vi "Model.vi"() -> ()   [LabVIEW 2016]
uses:
  <vilib>/Analysis/Matrix/Datatypes/RealMatrix.ctl
  Enum_activations.ctl
  <vilib>/Analysis/Matrix/NI_Matrix.lvlib
panel:
  out "Cost":dbl(graph)
  in  "Learning_Rate":dbl
  out "m":i32
  out "Costs":dbl[](array[numeric])
  in  "Y":T1
  in  "Parameters":T3(array[cluster])
  in  "Epochs":i32
  out "Predictions":T1
  in  "X":T1
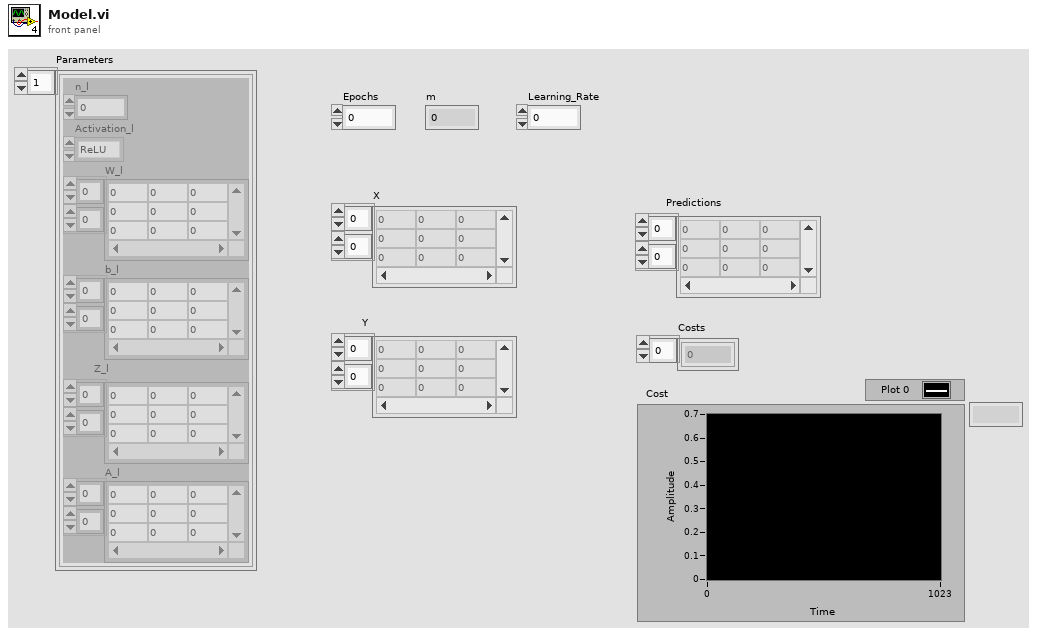
[diagram p1: front panel]
types:
  T1 = typedef "NI_Matrix.lvlib/RealMatrix.ctl" = dbl[][]
  T2 = typedef "Enum_activations.ctl" = enum16{"ReLU", "Sigmoid"}
  T3 = cluster{"n_l":i32, "Activation_l":T2, "W_l":T1, "b_l":T1, "Z_l":T1, "A_l":T1}[]
  T4 = cluster{"n_l":i32, "Activation_l":T2, "W_l":T1, "b_l":T1, "Z_l":T1, "A_l":T1}
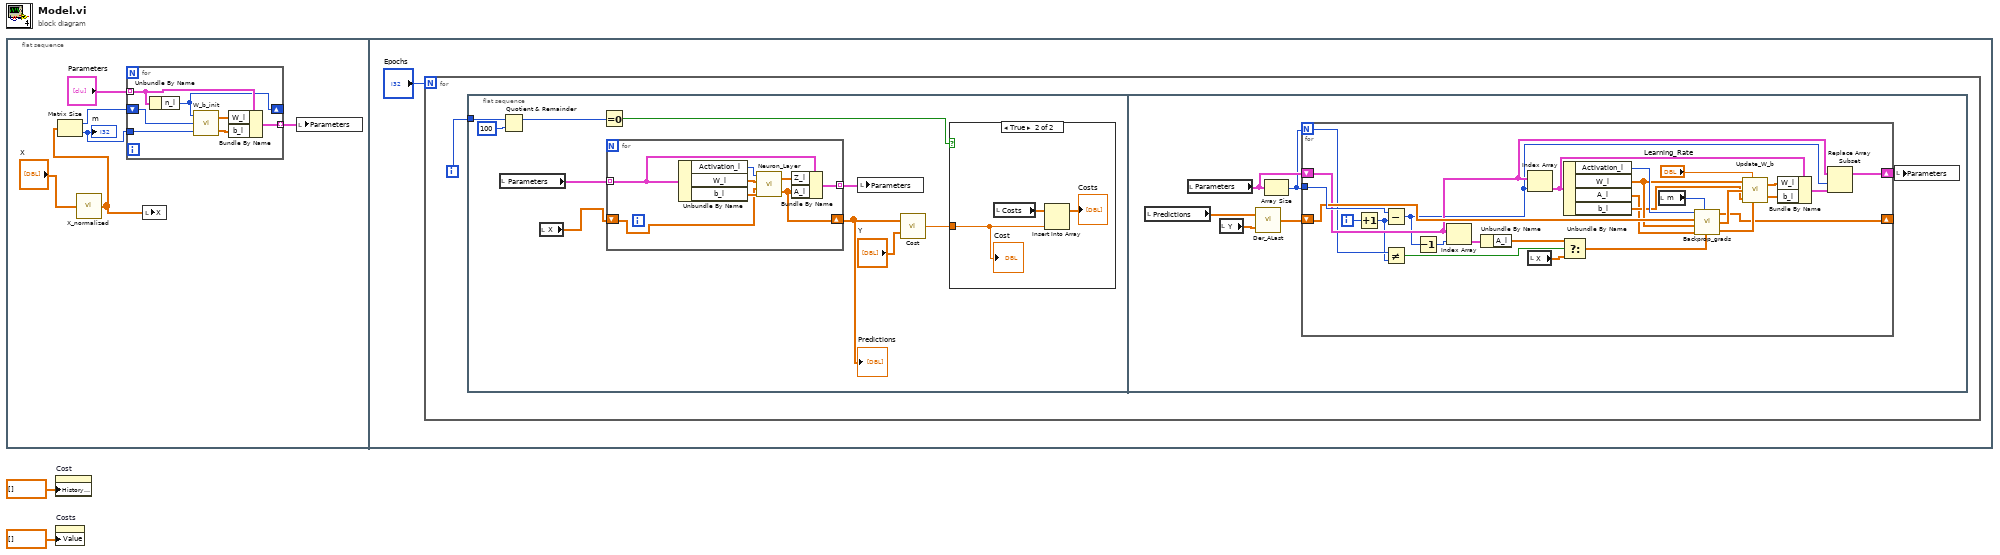
[diagram p0: block diagram]
diagram:
  n1 = flat-sequence {
    frame #0 {
      n2 = call "X_normalized.vi"("X"="X") -> ("X_normalized"=w3:T1)
      n3 = Matrix Size(0:w3) -> (1:w5:i32, 2:w6:i32)
      "m" <- w6
      n4 = for {
        tunnel: "Parameters" -> [w14] mode=indexing
        tunnel: w6 -> [w15]
        shift-right: [w10] -> _
        shift-left: w5 -> [w9]
        tunnel: [w11] -> w7 mode=indexing
        n5 = Unbundle By Name(w14) -> ("n_l"=w10:i32)
        n6 = call "W_b_init.vi"("m"=w15, "n_l-1"=w9, "n_l"=w10) -> ("b_l"=w12:T1, "W_l"=w13:T1)
        n7 = Bundle By Name(cluster=w14, "W_l"=w13, "b_l"=w12) -> (w11:T4)
      }
      n8 = local write "X"(w3) -> ()
      n9 = local write "Parameters"(w7) -> ()
    }
    frame #1 {
      n10 = for {
        N: "Epochs" -> [_]
        i -> [w17]
        n11 = flat-sequence {
          tunnel: w17 -> [w25]
          frame #0 {
            n12 = local read "Parameters"() -> (w27:T3)
            n13 = Quotient & Remainder(x=w25, y=100) -> (x-y*floor(x/y)=w23:i32)  [unwired: 1 out]
            n14 = local read "X"() -> (w18:T1)
            n15 = Equal To 0?(x=w23) -> (x = 0?=w22:bool)
            n16 = for {
              tunnel: w27 -> [w35] mode=indexing
              shift-right: [w33] -> w19
              shift-left: w18 -> [w31]
              tunnel: [w32] -> w20 mode=indexing
              n17 = Unbundle By Name(w35) -> ("Activation_l"=w38:T2, "W_l"=w37:T1, "b_l"=w36:T1)
              n18 = call "Neuron_Layer.vi"("b"=w36, "A_l-1"=w31, "W"=w37, "Activation"=w38) -> ("A_l"=w33:T1, "Z"=w34:T1)
              n19 = Bundle By Name(cluster=w35, "Z_l"=w34, "A_l"=w33) -> (w32:T4)
            }
            "Predictions" <- w19
            n20 = local write "Parameters"(w20) -> ()
            n21 = call "Cost.vi"("Y"="Y", "Predictions"=w19) -> ("Cost"=w21:dbl)
            n22 = case shown="True" w22 {
              tunnel: w21 -> [_ w28]
              frame False {
              }
              frame True {
                n23 = local read "Costs"() -> (w30:dbl[])
                n24 = Insert Into Array(array=w30, new element=w28) -> (→"Costs":dbl[])  [unwired: 1 in]
                "Cost" <- w28
              }
            }
          }
          frame #1 {
            n25 = local read "Predictions"() -> (w42:T1)
            n26 = local read "Parameters"() -> (w41:T3)
            n27 = local read "Y"() -> (w44:T1)
            n28 = call "Der_ALast.vi"("Y"=w44, "A_l"=w42) -> ("d_AL"=w43:T1)
            n29 = Array Size(array=w41) -> (size(s)=w40:i32)
            n30 = for {
              N: w40 -> [w53]
              shift-right: [w45] -> _
              shift-left: w43 -> [w68]
              tunnel: w40 -> [w71]
              shift-right: [w54] -> w39
              shift-left: w41 -> [w56]
              i -> [w52]
              n31 = Increment(x=w52) -> (x+1=w49:i32)
              n32 = Subtract(x=w71, y=w49) -> (x-y=w55:i32)
              n33 = Not Equal?(x=w53, y=w49) -> (x != y?=w51:bool)
              n34 = Decrement(x=w55) -> (x-1=w70:i32)
              n35 = Index Array(array=w56, index=w70) -> (element=w67:T4)
              n36 = Unbundle By Name(w67) -> ("A_l"=w47:T1)
              n37 = Index Array(array=w56, index=w55) -> (element=w60:T4)
              n38 = local read "X"() -> (w50:T1)
              n39 = Select(t=w47, s=w51, f=w50) -> (s? t:f=w46:T1)
              n40 = Unbundle By Name(w60) -> ("Activation_l"=w69:T2, "W_l"=w65:T1, "A_l"=w48:T1, "b_l"=w63:T1)
              n41 = local read "m"() -> (w66:i32)
              n42 = call "Backprop_grads.vi"("Activation"=w69, "m"=w66, "dA_l"=w68, "W_l"=w65, "A_l-1"=w46, "A_l"=w48) -> ("dA_l-1"=w45:T1, "dW_l"=w64:T1, "db_l"=w62:T1)
              n43 = call "Update_W_b.vi"("W_l"=w65, "Learning_Rate"="Learning_Rate", "dW_l"=w64, "b_l"=w63, "db_l"=w62) -> ("New_Wl"=w59:T1, "New_bl"=w58:T1)
              n44 = Bundle By Name(cluster=w60, "W_l"=w59, "b_l"=w58) -> (w57:T4)
              n45 = Replace Array Subset(array=w56, new element=w57, index=w55) -> (w54:T3)
            }
            n46 = local write "Parameters"(w39) -> ()
          }
        }
      }
    }
  }
  n47 = property on="Cost" class="WFChart (strict)"("History Data"=dbl[] []) -> ()  [unwired: 2 in, 2 out]
  n48 = property on="Costs" class="Arr (strict)"("Value"=dbl[] [] ("Costs")) -> ()  [unwired: 2 in, 2 out]
